vi "Basic Data Collection.vi"() -> ()   [LabVIEW 2020]
uses:
  instr.lib/Siemens ELAN/Message Header.ctl
  instr.lib/Siemens ELAN/Channel Status.ctl
  instr.lib/Siemens ELAN/Siemens ELAN.lvlib
panel:
  out "Numeric":i32
  out "Data Array":string[][](array[string])
  out "Message Header":T1 {"Source Address" format="%.0x"; "Target Address" format="%.0x"}
  in  "stop":bool
  in  "VISA resource name":refnum<visa-resource-name>="OXYMAT"
  out "error out":errorcluster
  in  "error in":errorcluster
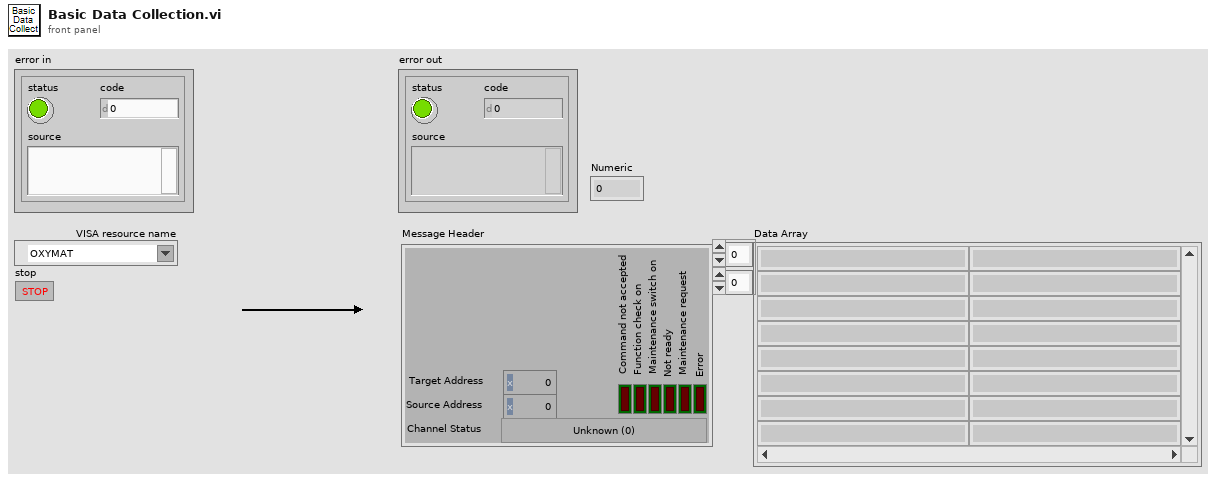
[diagram p1: front panel]
types:
  T1 = typedef "Siemens ELAN.lvlib/Message Header.ctl" = cluster{"Target Address":u8, "Source Address":u8, "Error":bool, "Maintenance request":bool, "Not ready":bool, "Maintenance switch on":bool, "Function check on":bool, "Command not accepted":bool, "Channel Status":T2}
  T2 = typedef "Siemens ELAN.lvlib/Channel Status.ctl" = enum8{"Unknown (0)", "Warm-up", "Pause", "Standby", "Measure", "Zero calibration", "Adjust component slope", "Unknown (7)", "Adjust curve dip", "Adjust linearization sensitivity", "Adjust temperature compensation", "Adjust pressure compensation", "Adjust linearization zero", "Adjust flow sensor", "Autocal", "Adjust phase", "Zero calibration of O2 sensor", "Synchronous zero calibration", "Purging for synchronous zero calibration", "Adjust analog output", "Adjust analog input", "Cleaning", "Unknown (>21)"}
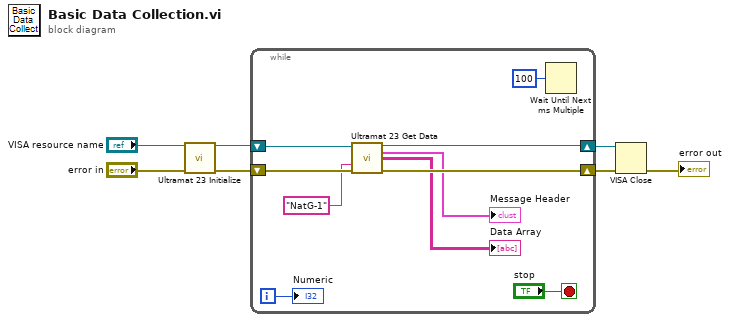
[diagram p0: block diagram]
diagram:
  n1 = call "Ultramat 23 Initialize.vi"("VISA resource name"="VISA resource name", "error in (no error)"="error in") -> ("VISA Session Out"=w6:refnum<visa-resource-name>, "error out"=w3:errorcluster)  [unwired: 8 in, 4 out]
  n2 = while {
    shift-right: [w16] -> w5
    shift-left: w6 -> [w17]
    shift-right: [w15] -> w4
    shift-left: w3 -> [w14]
    i -> [w8]
    stop <- "stop" stop-if-true
    n3 = call "Ultramat 23 Get Data.vi"("VISA resource name"=w17, "Gas selected"="NatG-1", "error in (no error)"=w14) -> ("VISA Session Out"=w16:refnum<visa-resource-name>, "Message Header"=→"Message Header":T1, "Data Array"=→"Data Array":string[][], "error out"=w15:errorcluster)  [unwired: 8 in, 1 out]
    n4 = Wait Until Next ms Multiple(millisecond multiple=u32 100) -> ()  [unwired: 1 out]
    "Numeric" <- w8
  }
  n5 = VISA Close(VISA resource name=w5, error in (no error)=w4) -> (error out=→"error out":errorcluster)
